vi "Write ADU Packet.vi"(8 "error in (no error)":errorcluster, 9 "Modbus data unit":refnum<class "Modbus Data Unit (PDU).lvclass">, 10 "network protocol":refnum<class "Network Protocol.lvclass">, 11 "ASCII transmission data unit in":refnum<class "ASCII Data Unit.lvclass">) -> (0 "error out":errorcluster, 2 "network protocol out":refnum<class "Network Protocol.lvclass">, 3 "ASCII transmission data unit out":refnum<class "ASCII Data Unit.lvclass">)   [LabVIEW 2020, in "SubVIs.lvlib" / "ASCII Data Unit.lvclass"]
uses:
  <vilib>/Modbus/subvis/Transmission Data Unit (ADU)/ASCII Data Unit/ASCII Data Unit.lvclass
  C:/builds/penguin/iak/lvdsc/trunk/20.0/lv/vi.lib/Modbus/subvis/Transmission Data Unit (ADU)/Serial Data Unit/Serial Data Unit.lvclass
  C:/builds/penguin/iak/lvdsc/trunk/20.0/lv/vi.lib/Modbus/subvis/Transmission Data Unit (ADU)/Transmission Data Unit/Transmission Data Unit.lvclass
  <vilib>/Modbus/subvis/Modbus Data Unit (PDU)/Modbus Data Unit (PDU).lvclass
  <vilib>/Modbus/subvis/Protocol/Interfaces/Network Protocol/Network Protocol.lvclass
  <vilib>/Modbus/subvis/Modbus Data Unit (PDU)/Modbus Data Unit (PDU).lvclass/Modbus Data Unit (PDU).ctl
  <vilib>/Modbus/subvis/Transmission Data Unit (ADU)/Serial Data Unit/Serial Data Unit.lvclass/Serial Data Unit.ctl
  <vilib>/Modbus/subvis/Transmission Data Unit (ADU)/Transmission Data Unit/Transmission Data Unit.lvclass/Transmission Data Unit.ctl
  <vilib>/Utility/error.llb/Error Cluster From Error Code.vi
  <vilib>/ErrorRing/Error Ring.xnode
  <vilib>/Modbus/subvis/Transmission Data Unit (ADU)/Serial Data Unit/Serial Data Unit.lvclass
  <vilib>/Modbus/subvis/Transmission Data Unit (ADU)/Transmission Data Unit/Transmission Data Unit.lvclass
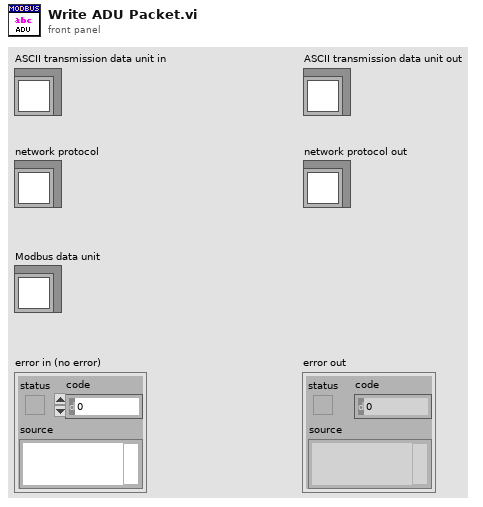
[diagram p1: front panel]
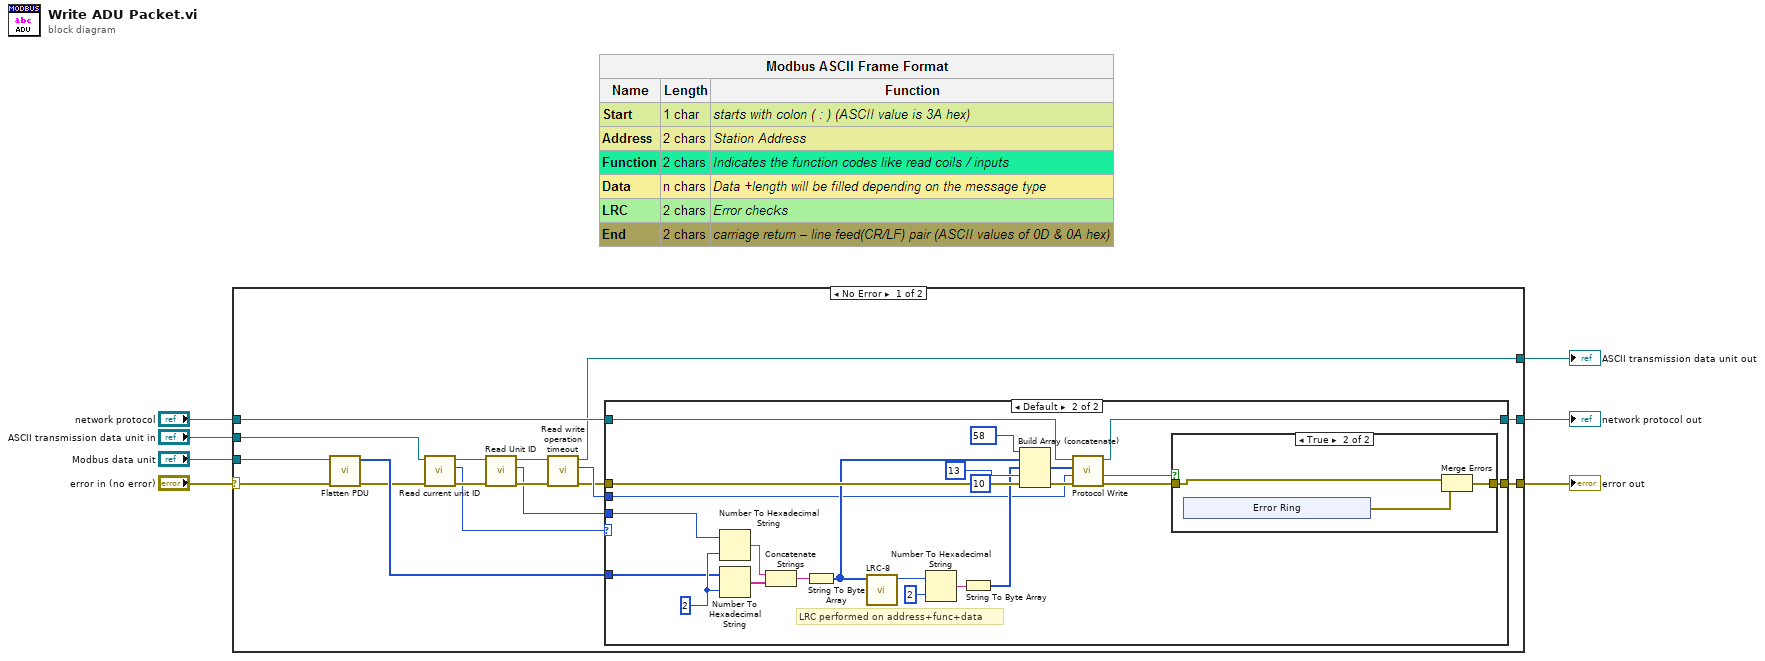
[diagram p0: block diagram]
diagram:
  n1 = case shown="No Error" "error in (no error)" {
    selector: "error in (no error)" -> [w23 w59]
    tunnel: [w20 w59] -> w4
    tunnel: "Modbus data unit" -> [w24 _]
    tunnel: "ASCII transmission data unit in" -> [w10 w57]
    tunnel: "network protocol" -> [w22 w58]
    tunnel: [w21 w58] -> w5
    tunnel: [w9 w57] -> w6
    frame No Error {
      n2 = call <vilib>:"Flatten PDU.vi"("error in (no error)"=w23, "Modbus data unit in"=w24) -> ("error out"=w11:errorcluster, "full Modbus data unit"=w19:u8[])  [unwired: 8 in]
      n3 = call <vilib>:"Read current unit ID.vi"("error in (no error)"=w11, "serial data unit in"=w10) -> ("error out"=w17:errorcluster, "request unit ID"=w12:u8, "serial data unit out"=w18:refnum<class "ASCII Data Unit.lvclass">)  [unwired: 7 in]
      n4 = call <vilib>:"Read Unit ID.vi"("error in"=w17, "transmission data unit in"=w18) -> ("error out"=w16:errorcluster, "unit ID"=w13:u8, "transmission data unit out"=w15:refnum<class "ASCII Data Unit.lvclass">)  [unwired: 7 in]
      n5 = call <vilib>:"Read write operation timeout.vi"("error in (no error)"=w16, "transmission data unit in"=w15) -> ("error out"=w8:errorcluster, "write operation timeout"=w14:i32, "transmission data unit out"=w9:refnum<class "ASCII Data Unit.lvclass">)  [unwired: 7 in]
      n6 = case shown="Default" w12 {
        tunnel: w22 -> [w25 w48]
        tunnel: [w25 w47] -> w21
        tunnel: [w26 w44] -> w20
        tunnel: w13 -> [_ w42]
        tunnel: w19 -> [_ w41]
        tunnel: w8 -> [w26 w35]
        tunnel: w14 -> [_ w27]
        frame 0 {
          # "request unit ID defaults to 1. If it is 0 it was set that way. If it was set that way, this is a slave trying to respond to a broadcast"
        }
        frame Default {
          w43 = 2
          # "LRC performed on address+func+data"
          n7 = Number To Hexadecimal String(1:w43, 2:w42) -> (0:w39:string)
          n8 = Number To Hexadecimal String(1:w43, 2:w41) -> (0:w40:string[])
          n9 = Concatenate Strings(w39, w40) -> (w29:string)
          n10 = String To Byte Array(string=w29) -> (unsigned byte array=w28:u8[])
          n11 = call <vilib>:"LRC-8.vi"("data"=w28) -> ("LRC-8"=w37:u8)  [unwired: 10 in]
          n12 = Number To Hexadecimal String(1:i16 2 ("width (-)"), 2:w37) -> (0:w31:string)
          n13 = String To Byte Array(string=w31) -> (unsigned byte array=w30:u8[])
          n14 = Build Array (concatenate)(u8 58 ("element"), w28, w30, u8 13 ("element"), u8 10 ("element")) -> (w36:u8[])
          n15 = call-dynamic "Protocol Write.vi"("error in (no error)"=w35, "timeout"=w27, "data"=w36, "protocol layer in"=w48) -> ("error out"=w45:errorcluster, "timed out?"=w46:bool, "protocol layer out"=w47:refnum<class "Network Protocol.lvclass">)  [unwired: 5 in]
          n16 = case shown="True" w46 {
            tunnel: w45 -> [w49 w51]
            tunnel: [w49 w52] -> w44
            frame False {
            }
            frame True {
              n17 = xnode "Error Ring"() -> ("error out"=w50:errorcluster)
              n18 = Merge Errors(w51, w50) -> (w52:errorcluster)
            }
          }
        }
      }
    }
    frame Error {
    }
  }
  "error out" <- w4
  "ASCII transmission data unit out" <- w6
  "network protocol out" <- w5
